vi "Put file.vi"(8 "error in (no error)":errorcluster, 9 "Local path":path, 10 "Remote path":string, 11 "SCP File Transfer in":refnum<class "SCP File Transfer.lvclass">) -> (0 "error out":errorcluster, 3 "SCP File Transfer out":refnum<class "SCP File Transfer.lvclass">)   [LabVIEW 2013, in "PL Framework Configuration Tool.lvlib" / "SCP File Transfer.lvclass"]
doc: "Puts the file located at \"Local path\" at \"Remote path\". The VI also creates all needed directories if the \"Remote path\" contains directories that don't exist on the target.\n\nThe recommended file path format for \"Remote path\" is \"/directory1/directory2/file.extension\". However, the VI will accept other formats and transform the path appropriately in most cases. Use the \"Strip path.vi\" and \"Build path.vi\" VIs to help with handling remote path strings."
uses:
  SCP File Transfer.lvclass
  SCP File Transfer.lvclass/SCP File Transfer.ctl
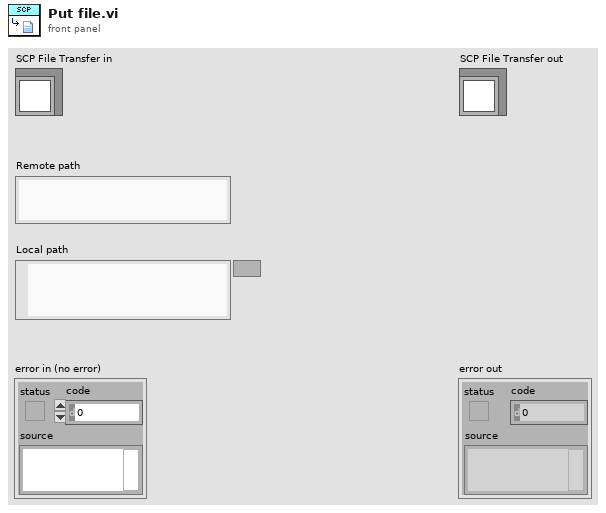
[diagram p1: front panel]
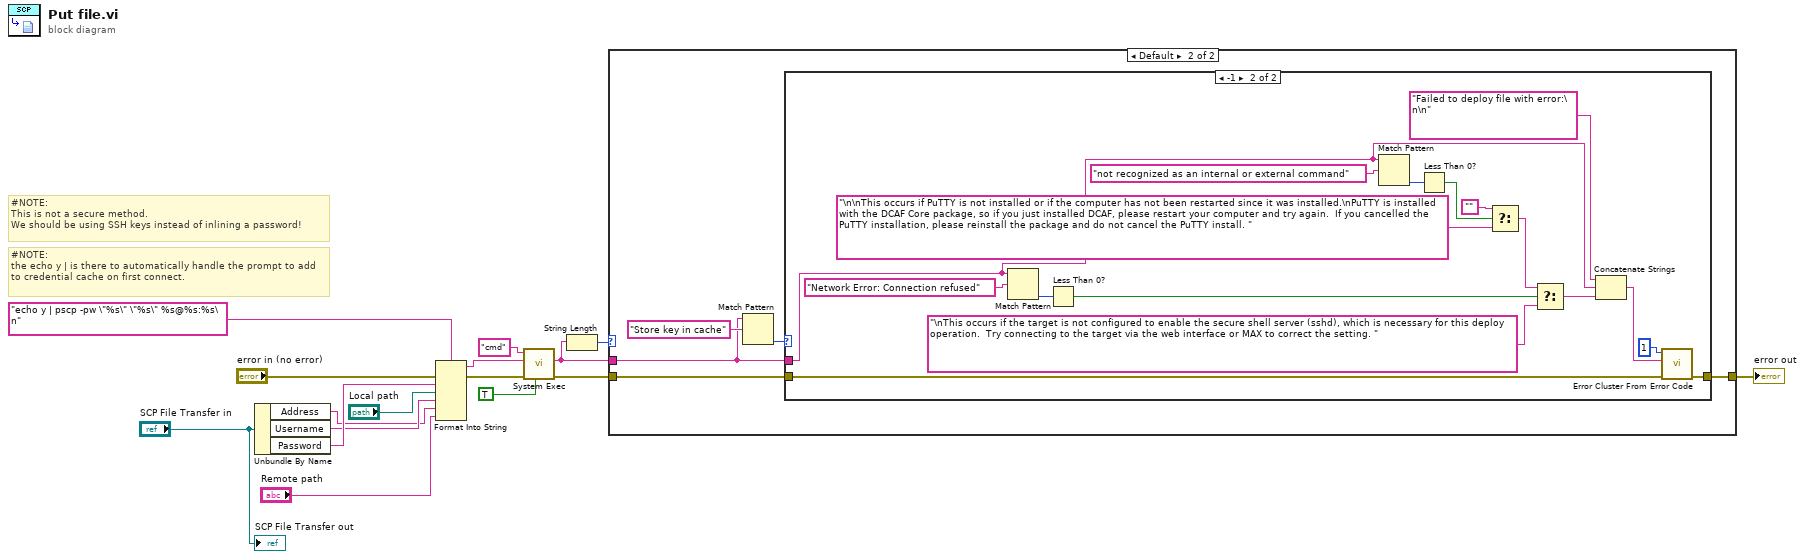
[diagram p0: block diagram]
diagram:
  # "#NOTE:\nthe echo y | is there to automatically handle the prompt to add to credential cache on first connect."
  # "#NOTE:\nThis is not a secure method.\nWe should be using SSH keys instead of inlining a password!"
  n1 = Unbundle By Name("SCP File Transfer in") -> ("Address"=w3:string, "Username"=w4:string, "Password"=w6:string)
  n2 = Format Into String(format string="echo y | pscp -pw \"%s\" \"%s\" %s@%s:%s\n", error in="error in (no error)", w6, "Local path", w4, w3, "Remote path") -> (resulting string=w7:string, error out=w14:errorcluster)  [unwired: 1 in]
  n3 = call <vilib>:"System Exec.vi"("run minimized? (F)"=TRUE, "error in (no error)"=w14, "standard input"=w7, "command line"="cmd") -> ("error out"=w9:errorcluster, "standard error"=w10:string)  [unwired: 4 in, 2 out]
  n4 = String Length(string=w10) -> (length=w11:i32)
  n5 = case shown="Default" w11 {
    tunnel: w10 -> [_ w19]
    tunnel: w9 -> [w17 w22]
    tunnel: [w17 w21] -> w8
    frame 0 {
    }
    frame Default {
      n6 = Match Pattern(string=w19, regular expression="Store key in cache") -> (offset past match=w18:i32)  [unwired: 1 in, 3 out]
      n7 = case shown="-1" w18 {
        tunnel: w22 -> [w23 w40]
        tunnel: [w23 w39] -> w21
        tunnel: w19 -> [_ w30]
        frame Default {
          # "This is an error message that is automatically handled by the 'echo y | prefix, due to the credentials for that target not being stored in the credential cache yet.  Don't scare a user with this expected error, suppress it and move on."
        }
        frame -1 {
          n8 = Match Pattern(string=w30, regular expression="Network Error: Connection refused") -> (offset past match=w28:i32)  [unwired: 1 in, 3 out]
          n9 = Less Than 0?(x=w28) -> (x < 0?=w27:bool)
          n10 = Match Pattern(string=w30, regular expression="not recognized as an internal or external command") -> (offset past match=w33:i32)  [unwired: 1 in, 3 out]
          n11 = Less Than 0?(x=w33) -> (x < 0?=w34:bool)
          n12 = Select(t="", s=w34, f="\n\nThis occurs if PuTTY is not installed or if the computer has not been restarted since it was installed.\nPuTTY is installed with the DCAF Core package, so if you just installed DCAF, please restart your computer and try again.  If you cancelled the PuTTY installation, please reinstall the package and do not cancel the PuTTY install. ") -> (s? t:f=w26:string)
          n13 = Select(t=w26, s=w27, f="\nThis occurs if the target is not configured to enable the secure shell server (sshd), which is necessary for this deploy operation.  Try connecting to the target via the web interface or MAX to correct the setting. ") -> (s? t:f=w24:string)
          n14 = Concatenate Strings("Failed to deploy file with error:\n\n" ("string"), w30, w24) -> (w37:string)
          n15 = call <vilib>:"Error Cluster From Error Code.vi"("error in (no error)"=w40, "error message (\"\")"=w37, "error code (0)"=1) -> ("error out"=w39:errorcluster)  [unwired: 6 in]
        }
      }
    }
  }
  "error out" <- w8
  "SCP File Transfer out" <- "SCP File Transfer in"
